vi "dotNETChart_Property_Chart_Wall_Transparency_Writevi.vi"(4 "error in (no error)":errorcluster, 5 "Value":i32, 6 "Container State":T9, 7 "Display State In":T1={"Chart Settings clstr"={"Enable Mouse Zoom (only works in 2D mode)"=TRUE, "Chart Wall Transparency Level"=37, "Chart Wall Colour"=0, "x axis label"="X axis title", "y axis label"="Y axis title", "Enable3D"=TRUE, "3D Settings"={"Inclination"=20, "LightStyle"=2, "Perspective"=4, "WallWidth"=5, "Rotation"=25}, "BackGradientStyle"=2, "SkinStyle"=1, "Chart Background Gradient Colour"=0, "Chart Border Colour"=0, "Palette"=12, "LegendStyle"=0, "ChartType"=[10, 13], "SeriesDataColour"=[]}} {"Chart Settings clstr"."ChartType" items=["Point", "FastPoint", "Bubble", "Line", "Spline", "StepLine", "FastLine", "Bar", "StackedBar", "StackedBar100", "Column", "StackedColumn", "StackedColumn100", "Area", "SplineArea", "StackedArea", "StackedArea100", "Pie", "Doughnut", "Stock", "Candlestick", "Range", "SplineRange", "RangeBar", "RangeColumn", "Radar", "Polar", "ErrorBar", "BoxPlot", "Renko", "ThreeLineBreak", "Kagi", "PointAndFigure", "Funnel", "Pyramid"]; "Chart Settings clstr"."LegendStyle" items=["Column", "Row", "Table"]; "Chart Settings clstr"."Palette" items=["None", "Bright", "Grayscale", "Excel", "Light", "Pastel", "EarthTones", "SemiTransparent", "Berry", "Chocolate", "Fire", "SeaGreen", "BrightPastel"]; "Chart Settings clstr"."SkinStyle" items=["None", "Emboss", "Raised", "Sunken", "FrameThin1", "FrameThin2", "FrameThin3", "FrameThin4", "FrameThin5", "FrameThin6", "FrameTitle1", "FrameTitle2", "FrameTitle3", "FrameTitle4", "FrameTitle5", "FrameTitle6", "FrameTitle7", "FrameTitle8"]; "Chart Settings clstr"."BackGradientStyle" items=["None", "LeftRight", "TopBottom", "Center", "DiagonalLeft", "DiagonalRight", "HorizontalCenter", "VerticalCenter"]; "Chart Settings clstr"."3D Settings"."LightStyle" items=["None", "Simplistic", "Realistic"]}) -> (0 "error out":errorcluster, 3 "Display State Out":T1={"Chart Settings clstr"={"Enable Mouse Zoom (only works in 2D mode)"=TRUE, "Chart Wall Transparency Level"=37, "Chart Wall Colour"=0, "x axis label"="X axis title", "y axis label"="Y axis title", "Enable3D"=TRUE, "3D Settings"={"Inclination"=20, "LightStyle"=2, "Perspective"=4, "WallWidth"=5, "Rotation"=25}, "BackGradientStyle"=2, "SkinStyle"=1, "Chart Background Gradient Colour"=0, "Chart Border Colour"=0, "Palette"=12, "LegendStyle"=0, "ChartType"=[10, 13], "SeriesDataColour"=[]}} {"Chart Settings clstr"."ChartType" items=["Point", "FastPoint", "Bubble", "Line", "Spline", "StepLine", "FastLine", "Bar", "StackedBar", "StackedBar100", "Column", "StackedColumn", "StackedColumn100", "Area", "SplineArea", "StackedArea", "StackedArea100", "Pie", "Doughnut", "Stock", "Candlestick", "Range", "SplineRange", "RangeBar", "RangeColumn", "Radar", "Polar", "ErrorBar", "BoxPlot", "Renko", "ThreeLineBreak", "Kagi", "PointAndFigure", "Funnel", "Pyramid"]; "Chart Settings clstr"."LegendStyle" items=["Column", "Row", "Table"]; "Chart Settings clstr"."Palette" items=["None", "Bright", "Grayscale", "Excel", "Light", "Pastel", "EarthTones", "SemiTransparent", "Berry", "Chocolate", "Fire", "SeaGreen", "BrightPastel"]; "Chart Settings clstr"."SkinStyle" items=["None", "Emboss", "Raised", "Sunken", "FrameThin1", "FrameThin2", "FrameThin3", "FrameThin4", "FrameThin5", "FrameThin6", "FrameTitle1", "FrameTitle2", "FrameTitle3", "FrameTitle4", "FrameTitle5", "FrameTitle6", "FrameTitle7", "FrameTitle8"]; "Chart Settings clstr"."BackGradientStyle" items=["None", "LeftRight", "TopBottom", "Center", "DiagonalLeft", "DiagonalRight", "HorizontalCenter", "VerticalCenter"]; "Chart Settings clstr"."3D Settings"."LightStyle" items=["None", "Simplistic", "Realistic"]})   [LabVIEW 2013, in "dotNETChart XControl.xctl"]
uses:
  dotNETChart XControl.xctl
  <vilib>/_xctls/Container State.ctl
  dotNETChart State 1.ctl
  typedefs/ChartSettings cluster.ctl
  typedefs/3DSettings.ctl
  typedefs/BackGradientStyle.ctl
  typedefs/SkinStyle.ctl
  typedefs/Palette.ctl
  typedefs/LegendStyle.ctl
  typedefs/ChartType.ctl
  <vilib>/_xctls/XControlSupport.lvlib
panel:
  # "Replace the Value Control below with a Control of desired type.\nDo not remove this Control or the others from the connector pane.\nDo not change the connector pane pattern.\nThe Value control should always be the third terminal from top on the input side in the connector pane."
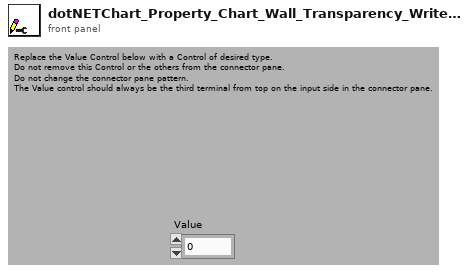
[diagram p1: front panel]
types:
  T1 = typedef "dotNETChart XControl.xctl/dotNETChart State 1.ctl" = cluster{"Chart Settings clstr":T2}
  T2 = typedef "ChartSettings cluster.ctl" = cluster{"Enable Mouse Zoom (only works in 2D mode)":bool, "Chart Wall Transparency Level":i32, "Chart Wall Colour":u32, "x axis label":string, "y axis label":string, "Enable3D":bool, "3D Settings":T3, "BackGradientStyle":T4, "SkinStyle":T5, "Chart Background Gradient Colour":u32, "Chart Border Colour":u32, "Palette":T6, "LegendStyle":T7, "ChartType":T8[], "SeriesDataColour":u32[]}
  T3 = typedef "3DSettings.ctl" = cluster{"Inclination":i32, "LightStyle":i32, "Perspective":i32, "WallWidth":i32, "Rotation":i32}
  T4 = typedef "BackGradientStyle.ctl" = i32
  T5 = typedef "SkinStyle.ctl" = i32
  T6 = typedef "Palette.ctl" = i32
  T7 = typedef "LegendStyle.ctl" = i32
  T8 = typedef "ChartType.ctl" = i32
  T9 = typedef "XControlSupport.lvlib/Container State.ctl" = cluster{"Indicator?":bool, "Run Mode?":bool, " Refnum":refnum<vi>}
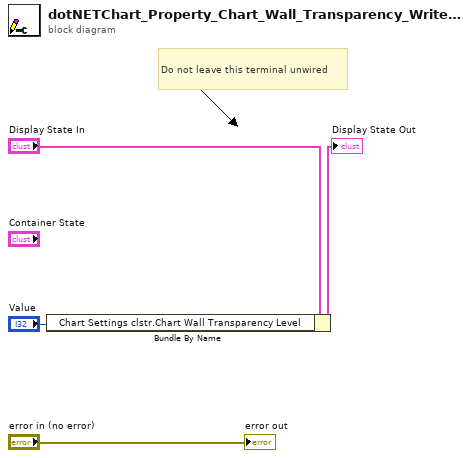
[diagram p0: block diagram]
diagram:
  # "Do not leave this terminal unwired"
  n1 = Bundle By Name(cluster="Display State In", "Chart Settings clstr.Chart Wall Transparency Level"="Value") -> (→"Display State Out":T1)
  "error out" <- "error in (no error)"
